vi "readRangeContinuousMillimeters.vi"(7 "io_timeout":u16, 8 "error in":errorcluster, 10 "Slave Address(7 bit)":u8, 11 "I2C Ref In":T1) -> (0 "error out":errorcluster, 1 "did_timeout":bool, 2 "Range":u16, 3 "I2C Ref Out":T1={"myRIO Reference"={"myRIO Model"=enum."Unknown", "myRIO Hardware Reference"={"Generic FPGA Reference"=refnum, "Allow multiple opens"=FALSE}}, "I2C Channels Enum"=enum."Not Connected", "I2C Configuration"={"I2C Transfer Rate"=enum."Fast mode (400 kbps)"}})   [LabVIEW 2018]
uses:
  <vilib>/myRIO/Instrument Drivers/Onboard IO/I2C/typedefs/I2C Reference.ctl
  <vilib>/myRIO/Common/Instrument Driver Framework/Utilities/typedefs/myRIO Generic Hardware Reference.ctl
  <vilib>/myRIO/Common/Instrument Driver Framework/Utilities/typedefs/Hardware Version Enum.ctl
  <vilib>/myRIO/Common/Instrument Driver Framework/Utilities/typedefs/myRIO v1.0 Reference.ctl
  <vilib>/myRIO/Common/Instrument Driver Framework/Utilities/typedefs/Generic FPGA Reference.ctl
  <vilib>/myRIO/Common/Instrument Driver Framework/myRIO v1.0/I2C/typedefs/I2C Channels Enum.ctl
  <vilib>/myRIO/Instrument Drivers/Onboard IO/I2C/typedefs/I2C Configuration.ctl
  <vilib>/myRIO/Instrument Drivers/Onboard IO/I2C/typedefs/I2C Transfer Rate.ctl
  <vilib>/Utility/error.llb/Error Cluster From Error Code.vi
  <vilib>/myRIO/Common/Instrument Driver Framework/myRIO v1.0/I2C/vis/myRIO v1.0 Write I2C.vi
  <vilib>/myRIO/Common/Instrument Driver Framework/myRIO v1.0/I2C/vis/myRIO v1.0 Read I2C.vi
  <vilib>/myRIO/Instrument Drivers/Onboard IO/I2C/I2C.lvlib
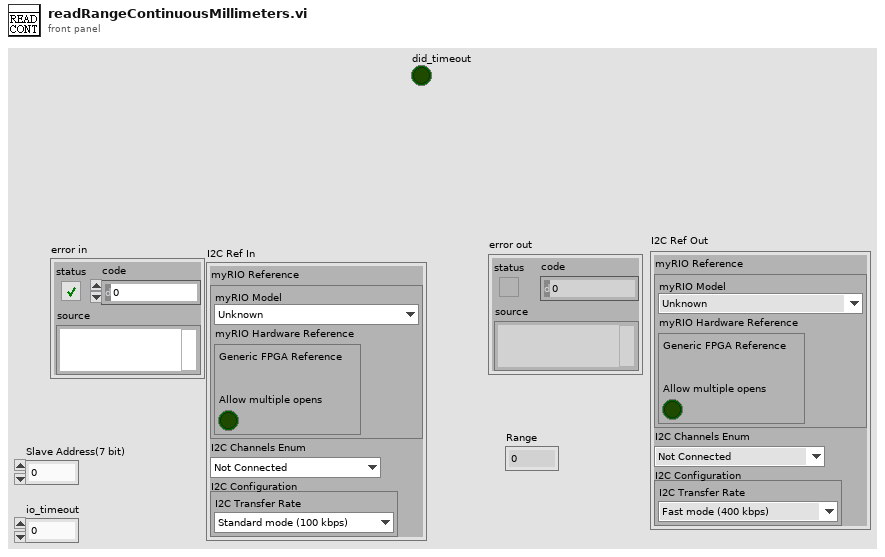
[diagram p1: front panel]
types:
  T1 = typedef "I2C.lvlib/I2C Reference.ctl" = cluster{"myRIO Reference":T2, "I2C Channels Enum":T6, "I2C Configuration":T7}
  T2 = typedef "myRIO Generic Hardware Reference.ctl" = cluster{"myRIO Model":T3, "myRIO Hardware Reference":T4}
  T3 = typedef "Hardware Version Enum.ctl" = enum16{"Unknown", "myRIO-1900", "myRIO-1950", "roboRIO", "NI ELVIS RIO CM", "ELVIS III"}
  T4 = typedef "myRIO v1.0 Reference.ctl" = cluster{"Generic FPGA Reference":T5, "Allow multiple opens":bool}
  T5 = typedef "Generic FPGA Reference.ctl" = refnum<k20>
  T6 = typedef "I2C Channels Enum.ctl" = enum16{"Not Connected", "A/I2C", "B/I2C", "I2C/I2C"}
  T7 = typedef "I2C.lvlib/I2C Configuration.ctl" = cluster{"I2C Transfer Rate":T8}
  T8 = typedef "I2C.lvlib/I2C Transfer Rate.ctl" = enum16{"Standard mode (100 kbps)", "Fast mode (400 kbps)"}
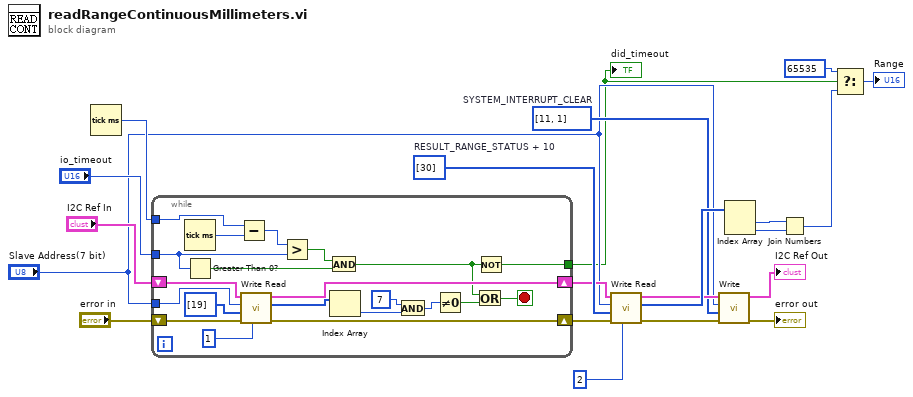
[diagram p0: block diagram]
diagram:
  w7 = u8[] [11, 1]  # SYSTEM_INTERRUPT_CLEAR
  w13 = u8[] [30]  # RESULT_RANGE_STATUS + 10
  n1 = Tick Count (ms)() -> (millisecond timer value=w21:u32)
  n2 = while {
    tunnel: "Slave Address(7 bit)" -> [w30]
    tunnel: w21 -> [w37]
    tunnel: "io_timeout" -> [w34]
    tunnel: [w24] -> w3
    shift-right: [w29] -> w14
    shift-left: "error in" -> [w27]
    shift-right: [w28] -> w12
    shift-left: "I2C Ref In" -> [w26]
    stop <- w31 stop-if-true
    n3 = Tick Count (ms)() -> (millisecond timer value=w36:u32)
    n4 = Greater Than 0?(x=w34) -> (x > 0?=w32:bool)
    n5 = Subtract(x=w37, y=w36) -> (x-y=w35:u32)
    n6 = call <vilib>:"Write Read.vi"("Byte Count"=u32 1, "error in (no error)"=w27, "Bytes to Write"=u8[] [19], "Slave Address (7-bit)"=w30, "I2C Ref In"=w26) -> ("error out"=w29:errorcluster, "Bytes Read"=w41:u8[], "I2C Ref Out"=w28:T1)  [unwired: 3 in]
    n7 = Greater?(x=w35, y=w34) -> (0:w33:bool)
    n8 = And(x=w33, y=w32) -> (x .and. y?=w22:bool)
    n9 = Index Array(array=w41) -> (element=w39:u8)  [unwired: 1 in]
    n10 = And(x=u8 7, y=w39) -> (x .and. y?=w38:u8)
    n11 = Not Equal To 0?(x=w38) -> (x != 0?=w23:bool)
    n12 = Or(x=w22, y=w23) -> (x .or. y?=w31:bool)
    n13 = Not(x=w22) -> (.not. x?=w24:bool)
  }
  "did_timeout" <- w3
  n14 = call <vilib>:"Write Read.vi"("Byte Count"=u32 2, "error in (no error)"=w14, "Bytes to Write"=w13, "Slave Address (7-bit)"="Slave Address(7 bit)", "I2C Ref In"=w12) -> ("error out"=w8:errorcluster, "Bytes Read"=w16:u8[], "I2C Ref Out"=w9:T1)  [unwired: 3 in]
  n15 = call <vilib>:"Write.vi"("error in (no error)"=w8, "Bytes to Write"=w7, "Slave Address (7-bit)"="Slave Address(7 bit)", "I2C Ref In"=w9) -> ("error out"=→"error out":errorcluster, "I2C Ref Out"=→"I2C Ref Out":T1)  [unwired: 6 in]
  n16 = Index Array(array=w16) -> (element #1=w17:u8, element #2=w18:u8)  [unwired: 2 in]
  n17 = Join Numbers(hi=w17, lo=w18) -> ((hi.lo)=w2:u16)
  n18 = Select(t=u16 65535, s=w3, f=w2) -> (s? t:f=→"Range":u16)
